vi "Destructor.vi"(8 "error in":errorcluster, 11 "Detector in":refnum<class "PID.lvclass">) -> (0 "error out":errorcluster, 3 "Detector out":refnum<class "PID.lvclass">)   [LabVIEW 2011, in "PID.lvclass"]
doc: "Shutdown of the spectral detector and release of software resourses allocated to the detector."
uses:
  PID.lvclass
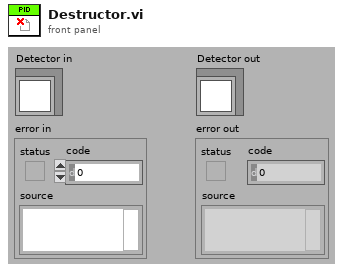
[diagram p1: front panel]
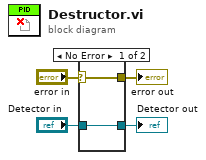
[diagram p0: block diagram]
diagram:
  n1 = case shown="No Error" "error in" {
    selector: "error in" -> [w5 w8]
    tunnel: [w5 w8] -> w3
    tunnel: [w6 w7] -> w1
    tunnel: "Detector in" -> [w6 w7]
    frame No Error {
    }
    frame Error {
    }
  }
  "error out" <- w3
  "Detector out" <- w1
